vi "game_of_life.vi"() -> ()   [LabVIEW 2020]
panel:
  out "game_of_life":cluster{"x_data":dbl[], "y_data":dbl[]}[](graph)
  out "generation":u32 caption="Generation"
  in  "update_interval_msec":u32 caption="Update interval (msec)"
  in  "height":u32 caption="Board height"
  in  "width":u32 caption="Board width"
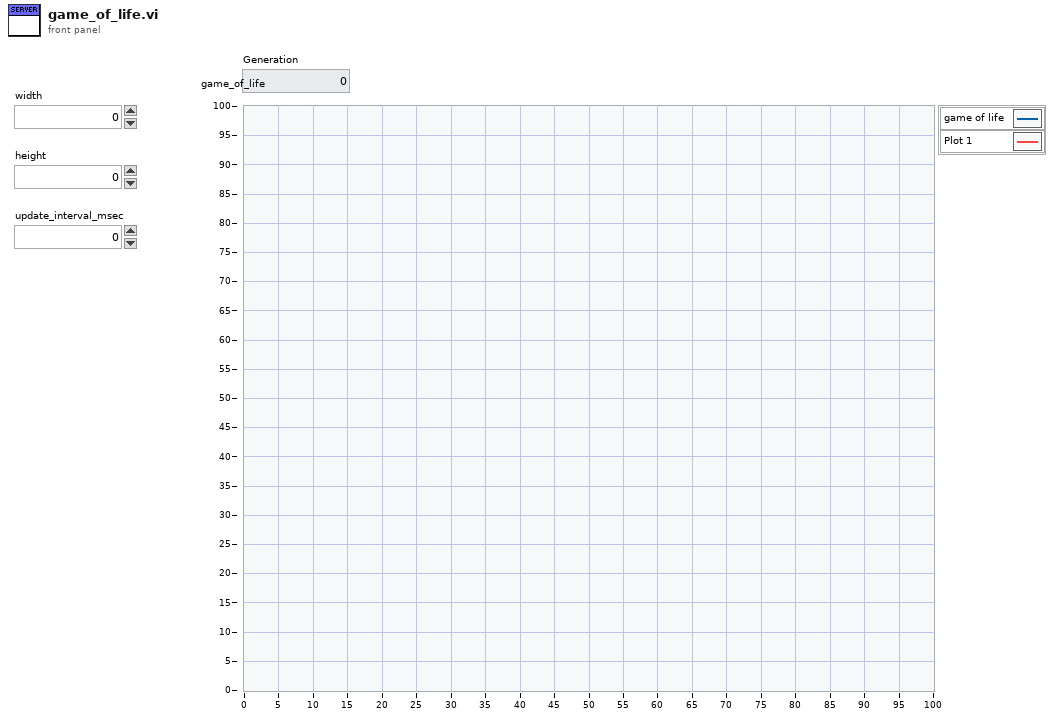
[diagram p1: front panel]
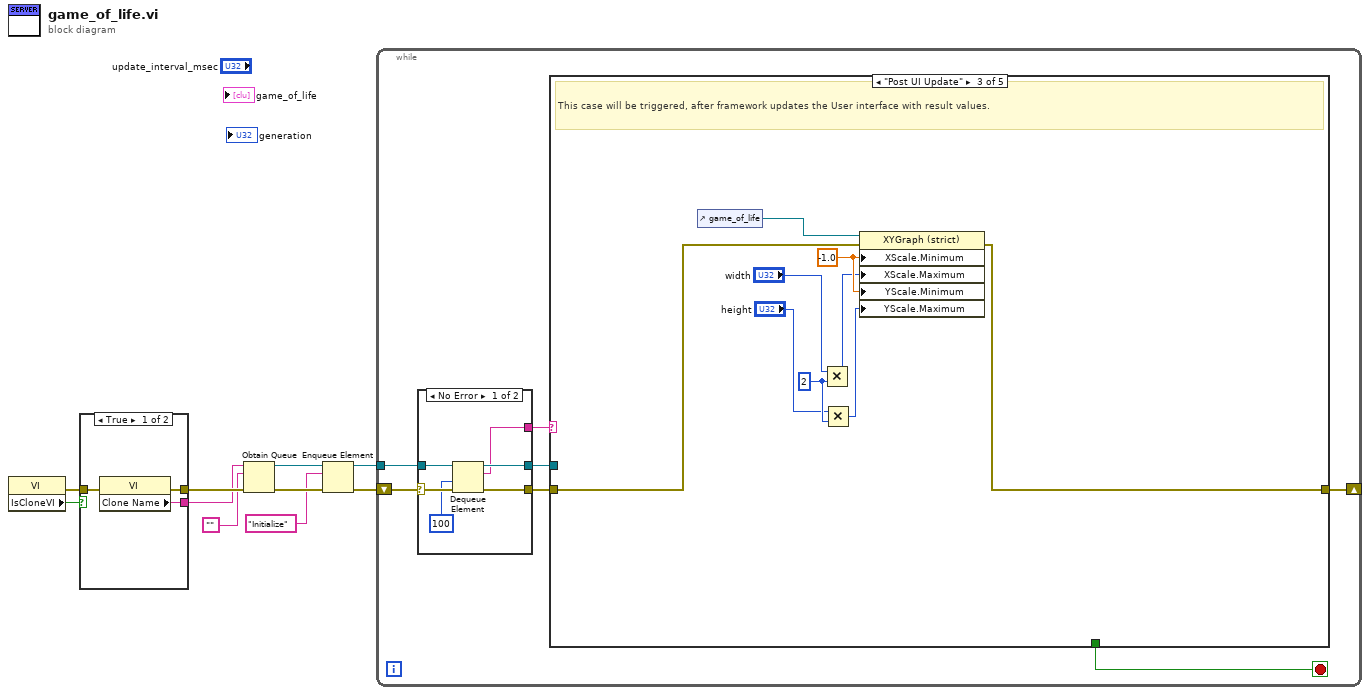
[diagram p0: block diagram]
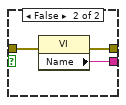
[diagram p2: hidden frame]
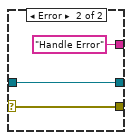
[diagram p3: hidden frame]
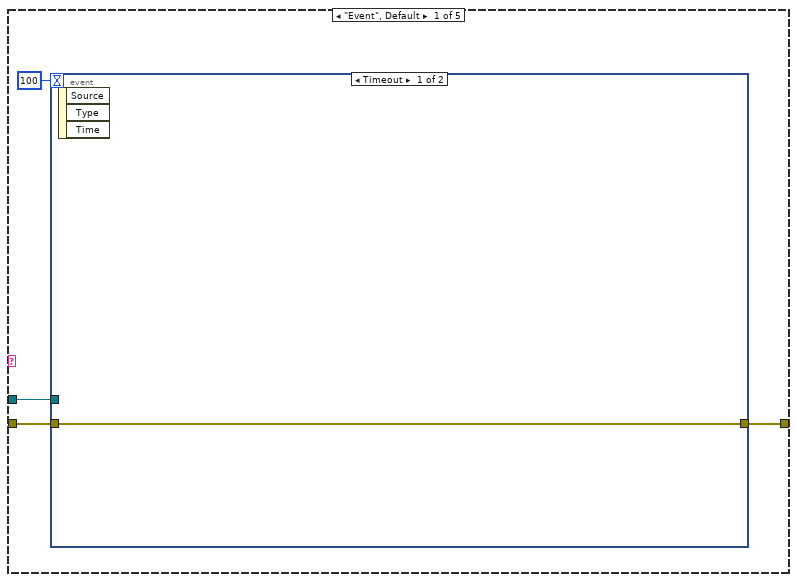
[diagram p4: hidden frame]
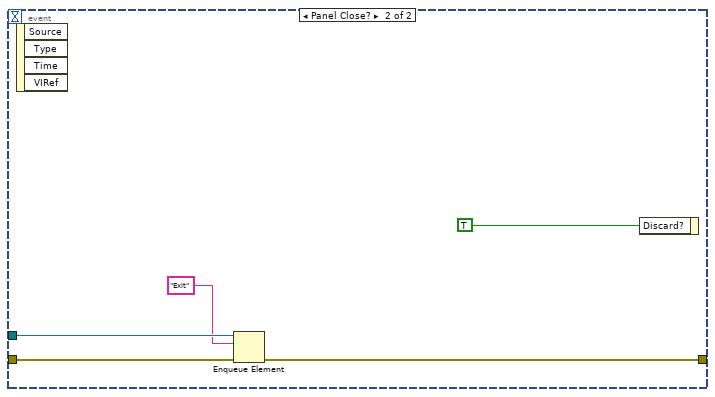
[diagram p5: hidden frame]
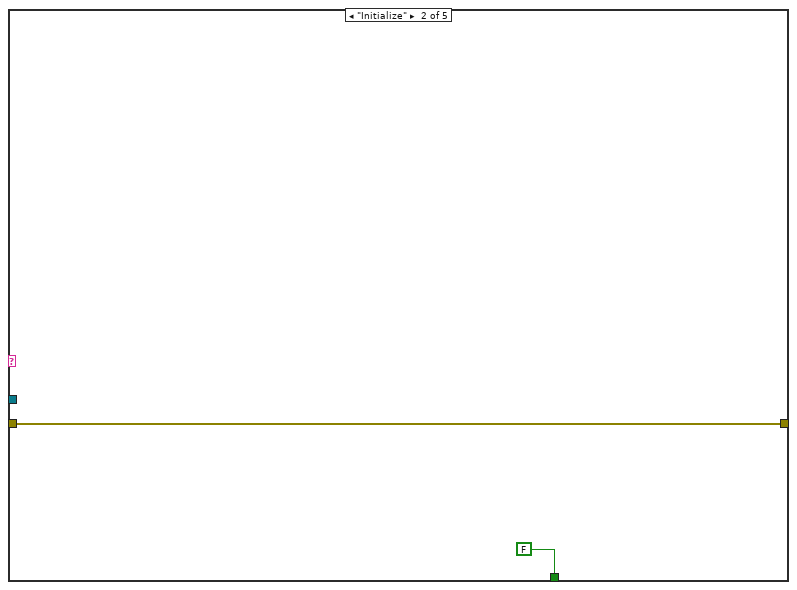
[diagram p6: hidden frame]
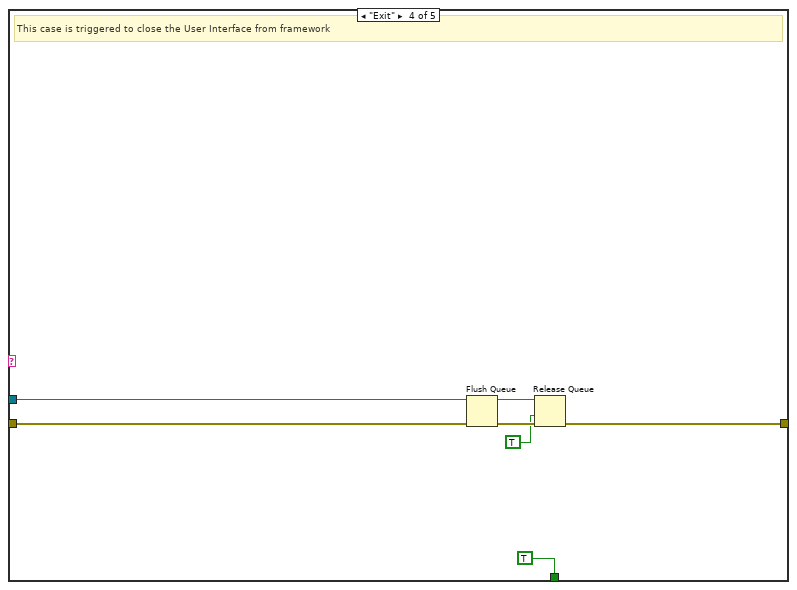
[diagram p7: hidden frame]
diagram:
  n1 = property class="VI"() -> (error out=w1:errorcluster, "IsCloneVI"=w2:bool)  [unwired: 2 in, 1 out]
  n2 = case shown="True" w2 {
    tunnel: [w13 w16] -> w10
    tunnel: [w12 w15] -> w9
    tunnel: w1 -> [w11 w14]
    frame True {
      n3 = property class="VI"(error in=w11) -> (error out=w13:errorcluster, "Clone Name"=w12:string)  [unwired: 1 in, 1 out]
    }
    frame False {
      n4 = property class="VI"(error in=w14) -> (error out=w16:errorcluster, "Name"=w15:string)  [unwired: 1 in, 1 out]
    }
  }
  n5 = Obtain Queue(name (unnamed)=w9, element data type="", error in (no error)=w10) -> (queue out=w6:refnum<queue>, error out=w8:errorcluster)  [unwired: 2 in, 1 out]
  n6 = Enqueue Element(queue=w6, element="Initialize", error in (no error)=w8) -> (queue out=w5:refnum<queue>, error out=w7:errorcluster)  [unwired: 1 in, 1 out]
  n7 = while {
    shift-right: [w18] -> _
    shift-left: w7 -> [w23]
    tunnel: w5 -> [w21]
    stop <- w17 stop-if-true
    n8 = case shown="No Error" w23 {
      selector: w23 -> [w29 w32]
      tunnel: [w28 w32] -> w22
      tunnel: w21 -> [w27 w31]
      tunnel: [w26 w31] -> w20
      tunnel: [w25 "Handle Error"] -> w19
      frame No Error {
        n9 = Dequeue Element(queue=w27, timeout in ms (-1)=100, error in (no error)=w29) -> (queue out=w26:refnum<queue>, element=w25:string, error out=w28:errorcluster)  [unwired: 1 out]
      }
      frame Error {
      }
    }
    n10 = case shown="\"Post UI Update\"" w19 {
      tunnel: w22 -> [w35 w43 w52 w60 w61]
      tunnel: w20 -> [w33 _ _ w58 _]
      tunnel: [w36 w43 w51 w55 w61] -> w18
      tunnel: [_ FALSE _ TRUE _] -> w17
      frame "Event", Default {
        n11 = event shown="[0] Timeout" {
          selector: _ -> [_ _]
          dyn-events: _ -> [_ _]
          timeout: 100 -> [_ _]
          tunnel: [w37 w40] -> w36
          tunnel: w35 -> [w37 w41]
          tunnel: w33 -> [_ w39]
          event Timeout {
            n12 = event-data() -> ()  [unwired: 1 in, 3 out]
          }
          event Panel Close? {
            n13 = event-data() -> ()  [unwired: 1 in, 4 out]
            n14 = Enqueue Element(queue=w39, element="Exit", error in (no error)=w41) -> (error out=w40:errorcluster)  [unwired: 1 in, 2 out]
            n15 = event-data("Discard?"=TRUE) -> ()  [unwired: 1 in, 1 out]
          }
        }
      }
      frame "Initialize" {
      }
      frame "Post UI Update" {
        w48 = u32 2 ("y")
        w53 = -1.0 ("X Scale.Range:Minimum")
        # "This case will be triggered, after framework updates the User interface with result values."
        n16 = control-ref of="game_of_life"() -> (w50:refnum<vi>)
        n17 = Multiply(x="width", y=w48) -> (x*y=w47:u32)
        n18 = Multiply(x="height", y=w48) -> (x*y=w45:u32)
        n19 = property on="Property Node" class="XYGraph (strict)"(reference=w50, error in=w52, "XScale.Minimum"=w53, "XScale.Maximum"=w47, "YScale.Minimum"=w53, "YScale.Maximum"=w45) -> (error out=w51:errorcluster)  [unwired: 1 out]
      }
      frame "Exit" {
        # "This case is triggered to close the User Interface from framework"
        n20 = Flush Queue(queue=w58, error in (no error)=w60) -> (queue out=w57:refnum<queue>, error out=w56:errorcluster)  [unwired: 1 out]
        n21 = Release Queue(queue=w57, force destroy? (F)=TRUE, error in (no error)=w56) -> (error out=w55:errorcluster)  [unwired: 2 out]
      }
      frame "Handle Error" {
      }
    }
  }
